vi "ZY to Y.vi"(10 "ZY_control":T3 {"Y_H" step=1.0; "SP" step=0.01 format="%.2f"}, 11 "Z_ASetState":T2) -> (2 "Z_control":T1={"Z_HSw"=1, "Z_HSetState"=enum."on", "Z_ASetState"=enum."on", "Z_DSetState"=enum."on"})   [LabVIEW 2019, in "Heating.lvlib"]
uses:
  ctl/ZY_control.ctl
  ctl/Z_State.ctl
  ctl/Y_state.ctl
  ctl/Z_control.ctl
  Heating.lvlib
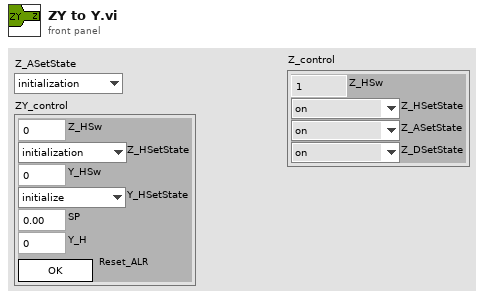
[diagram p1: front panel]
types:
  T1 = typedef "Heating.lvlib/Z_control.ctl" = cluster{"Z_HSw":u8, "Z_HSetState":T2, "Z_ASetState":T2, "Z_DSetState":T2}
  T2 = typedef "Heating.lvlib/Z_State.ctl" = enum8{"initialization", "alarm", "disabled", "not ready", "stop ready", "reserv", "switched off", "reserv2", "switched on", "check", "on min", "decrease out", "on", "increase out", "on max"}
  T3 = typedef "Heating.lvlib/ZY_control.ctl" = cluster{"Z_HSw":u8, "Z_HSetState":T2, "Y_HSw":u8, "Y_HSetState":T4, "SP":dbl, "Y_H":dbl, "Reset_ALR":bool}
  T4 = typedef "Heating.lvlib/Y_state.ctl" = enum8{"initialize", "alarm", "min", "stop", "hand", "auto", "max"}
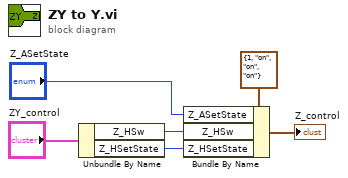
[diagram p0: block diagram]
diagram:
  n1 = Unbundle By Name("ZY_control") -> ("Z_HSw"=w2:u8, "Z_HSetState"=w3:T2)
  n2 = Bundle By Name(cluster=T1 {"Z_HSw"=1, "Z_HSetState"=enum."on", "Z_ASetState"=enum."on", "Z_DSetState"=enum."on"} ("Z_control"), "Z_ASetState"="Z_ASetState", "Z_HSw"=w2, "Z_HSetState"=w3) -> (→"Z_control":T1)
